vi "GetNumberOfSlots.vi"(11 "Chassis Cfg":refnum<class "ChassisCfg.lvclass">) -> (3 "# of Slots":i32)   [LabVIEW 2012, in "Configuration Grandmaster.lvlib" / "ChassisCfg.lvclass"]
uses:
  ChassisCfg.lvclass
  ChassisCfg.lvclass/ChassisCfg.ctl
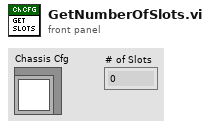
[diagram p1: front panel]
types:
  T1 = typedef "Chassis Type.ctl" = enum16{"Not Supported", "C Series 1-Slot", "C Series 4-Slot", "C Series 8-Slot", "PXI 8-Slot", "PXIe 18-Slot"}
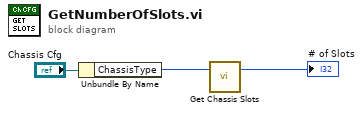
[diagram p0: block diagram]
diagram:
  n1 = Unbundle By Name("Chassis Cfg") -> ("ChassisType"=w2:T1)
  n2 = call "Get Chassis Slots.vi"("ChassisType"=w2) -> ("Num of Slots"=→"# of Slots":i32)  [unwired: 2 in]
